vi "Simultaneous Standard.vi"(0 "data server address":string="calcium", 1 "Uncalibrated Index":u32, 2 "Ports":T13) -> ()   [LabVIEW 2012]
uses:
  DAQ configuration/Sensor array.ctl
  DAQ configuration/channel identifier.ctl
  DAC apps/support/method.ctl
  DataServer/command cluster.ctl
  DataServer/command.ctl
  DAC apps/support/Daq state.ctl
  toolbar icons/simultaneous standard cal.ctl
  calib array.ctl
  conversion.ctl
  DAQ configuration/scale type.ctl
  correspondence table.ctl
  pH/pH scale.ctl
  Dissolved Oxygen/DO scale.ctl
  toolbar icons/Save calibration.ctl
  global scale array.vi
panel:
  out "Calibration Graph":cluster{dbl[], dbl[]}[](graph)
  in  "Number of Segments":i32=50
  in  "Save calibration":T1
  out "initial Calibration matrix":T2 {"D.O."."K" format="%.6f"; "D.O."."Temperature" format="%.2f"; "pH scale"."Buffers"."V/T" format="%.5f"; "pH scale"."Buffers"."Buffer" format="%.2f"; "pH scale"."Temperature" format="%.2f"; "offset (physical units)" format="%.5f"; "correspondence table"."volts" format="%.4f"; "correspondence table"."physical units" format="%.4f"; "second channel" min=-1; "offset (volts)" format="%.5f"; "conversion matrix" format="%.4e"}
  in  "Cancel Button":bool
  in  "new daq state":T8
  in  "Acquire Sample":T9
  out "daq state":T8
  in  "Stop acquisition":bool
  in  "Smoothed data frequency":ext=10.0 format="%.4f"
  out "Sampling data frequency":dbl
  in  "method":T10={"sampling interval"=0.1, "samples to average"=1, "data interval"=0.0, "stream data"=FALSE, "file path"=refnum, "command"={"command"=enum."Idle", "start time (ms)"=0, "Channel Indices"=[], "Scans per Sample"=1}} {"command"."Scans per Sample" min=1; "data interval" format="%.2f"; "samples to average" min=1 step=1; "sampling interval" format="%.2f"}
  out "chart":sgl[][](graph)
  out "backlog":u32
  in  "data points to acquire":u32=1000 min=1
  out "error":errorcluster={"status"=FALSE, "code"=56, "source"="TCP Read in \u0000TCP read variable.vi->read Volts data fast.vi->Signal Monitor"}
  in  "OK":bool
  out "units":string
  out "name":string
  in  "Standard\nChannel":i32 min=0 step=1
  # "C"
  # "kPa"
  # "C"
  # "s"
  # "s"
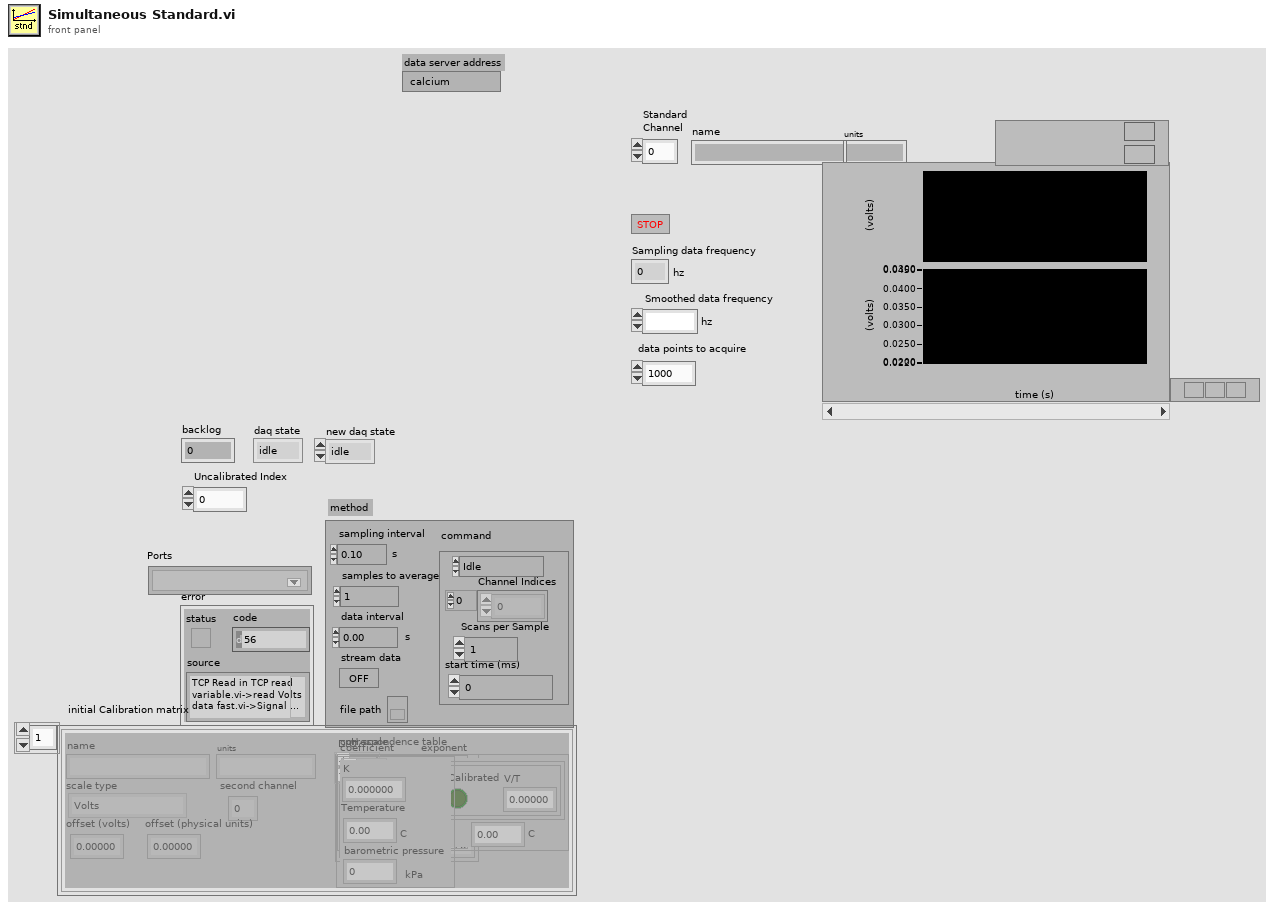
[diagram p1: front panel]
types:
  T1 = typedef "Save calibration.ctl" = bool
  T2 = typedef "calib array.ctl" = T3[]
  T3 = typedef "conversion.ctl" = cluster{"conversion matrix":sgl[][], "units":string, "name":string, "scale type":T4, "offset (volts)":dbl, "second channel":i8, "correspondence table":T5, "offset (physical units)":dbl, "pH scale":T6, "D.O.":T7}
  T4 = typedef "scale type.ctl" = enum16{"Volts", "Polynomial", "Correspondence Table", "pH", "Dissolved Oxygen", "Quadratic"}
  T5 = typedef "correspondence table.ctl" = cluster{"physical units":dbl, "volts":dbl}[]
  T6 = typedef "pH scale.ctl" = cluster{"Buffers":cluster{"Buffer":dbl, "Calibrated":bool, "V/T":dbl}[], "Temperature":dbl}
  T7 = typedef "DO scale.ctl" = cluster{"Temperature":dbl, "K":dbl, "barometric pressure":dbl}
  T8 = typedef "Daq state.ctl" = enum16{"idle", "start", "stream", "clear", "process data", "quit"}
  T9 = typedef "simultaneous standard cal.ctl" = bool
  T10 = typedef "method.ctl" = cluster{"sampling interval":sgl, "samples to average":u32, "data interval":sgl, "stream data":bool, "file path":refnum<file>, "command":T11}
  T11 = typedef "command cluster.ctl" = cluster{"command":T12, "start time (ms)":u32, "Channel Indices":i32[], "Scans per Sample":i32}
  T12 = typedef "command.ctl" = enum16{"Idle", "Send Data", "Send 1 Scan", "Logoff"}
  T13 = typedef "Sensor array.ctl" = T14[]
  T14 = typedef "channel identifier.ctl" = u16
  T15 = enum16{"Idle", "Send Data", "Send 1 Scan", "Logoff"}
  T16 = enum16{"Volts", "Polynomial", "Correspondence Table", "pH", "Dissolved Oxygen"}
  T17 = typedef "Server stats.ctl" = cluster{"scan rate":dbl, "# connections":i32, "channel settings":cluster{"Name":string, "upper input limits":sgl, "lower input limits":sgl, "Location":string}[]}
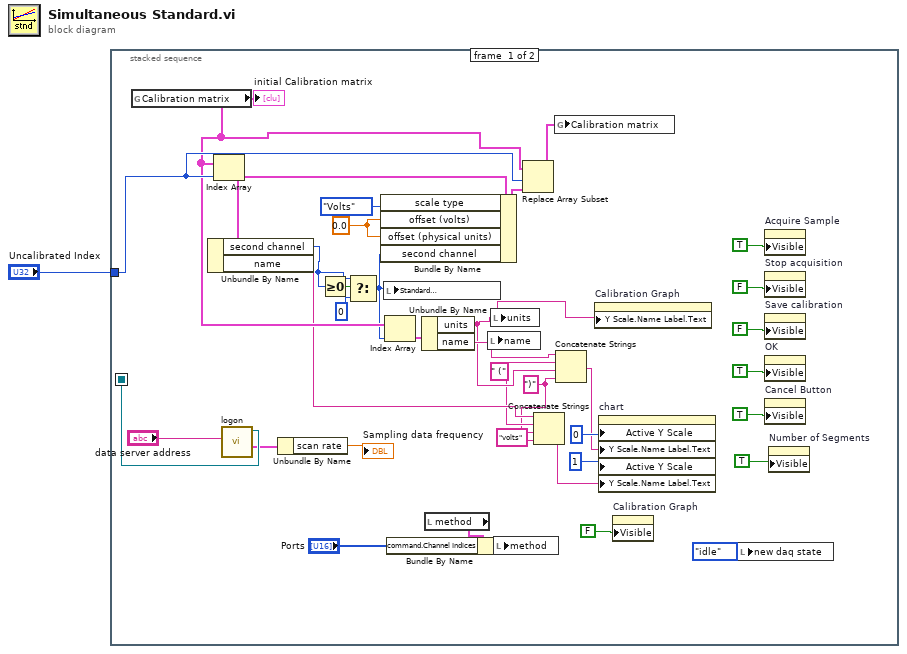
[diagram p0: block diagram]
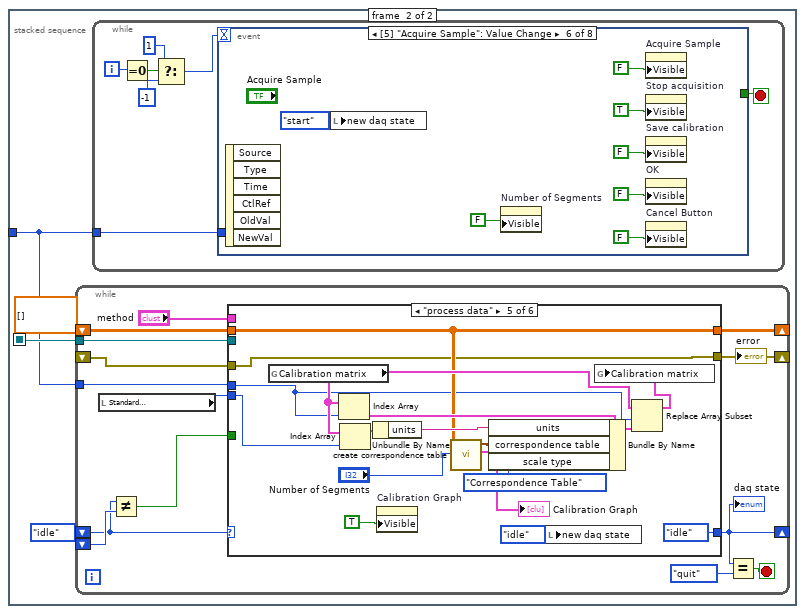
[diagram p2: hidden frame]
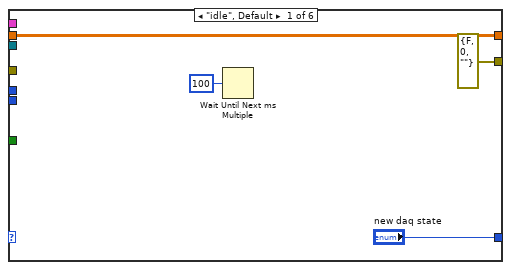
[diagram p3: hidden frame]
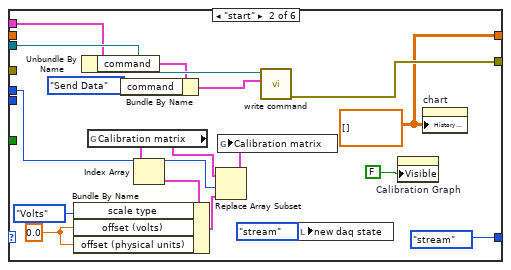
[diagram p4: hidden frame]
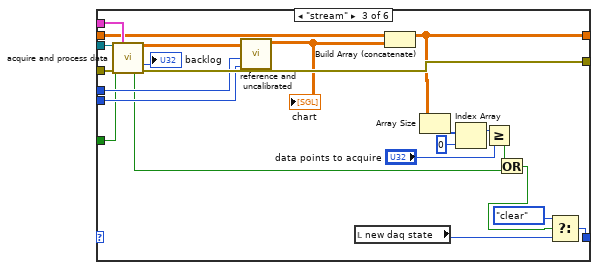
[diagram p5: hidden frame]
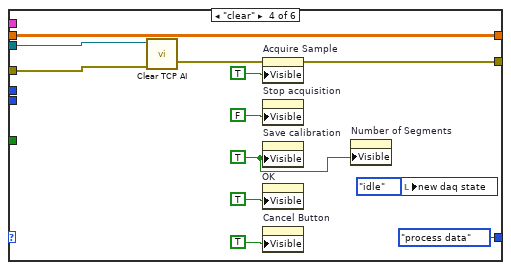
[diagram p6: hidden frame]
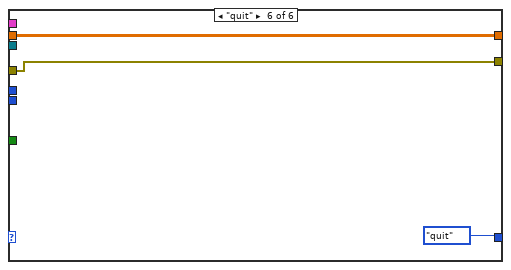
[diagram p7: hidden frame]
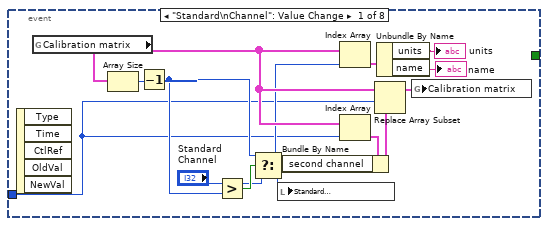
[diagram p8: hidden frame]
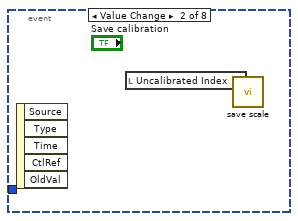
[diagram p9: hidden frame]
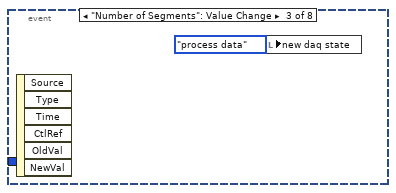
[diagram p10: hidden frame]
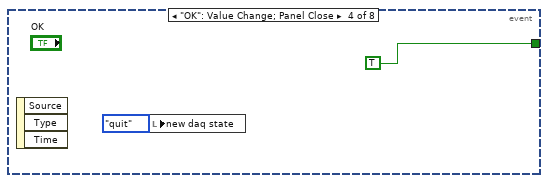
[diagram p11: hidden frame]
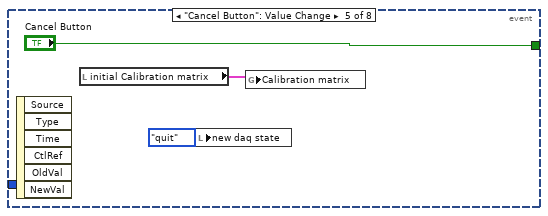
[diagram p12: hidden frame]
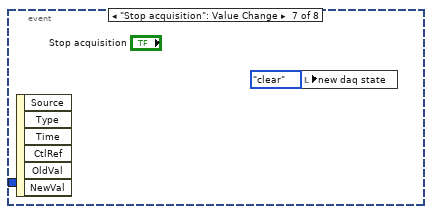
[diagram p13: hidden frame]
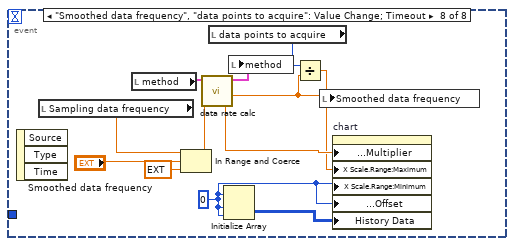
[diagram p14: hidden frame]
diagram:
  n1 = stacked-sequence {
    seq-local: [w5 _] -> [_ w42]
    tunnel: "Uncalibrated Index" -> [w29 w39]
    frame #0 {
      w8 = ")"
      w10 = " ("
      w27 = 0.0 ("offset (volts)")
      n2 = global read "global scale array.vi" "Calibration matrix"() -> (w22:T2)
      "initial Calibration matrix" <- w22
      n3 = Index Array(array=w22, index=w29) -> (element=w21:T3)
      n4 = Unbundle By Name(w21) -> ("second channel"=w20:i8, "name"=w11:string)
      n5 = call "logon.vi"("data server address in"="data server address") -> ("Server stats"=w4:T17, "connection ID"=w5:refnum<k5>)  [unwired: 7 in, 2 out]
      n6 = Unbundle By Name(w4) -> ("scan rate"=→"Sampling data frequency":dbl)
      n7 = Greater Or Equal To 0?(x=w20) -> (x >= 0?=w18:bool)
      n8 = Select(t=w20, s=w18, f=i8 0 ("second channel")) -> (s? t:f=w19:i8)
      n9 = Bundle By Name(cluster=w21, "scale type"=scale_type."Volts", "offset (volts)"=w27, "offset (physical units)"=w27, "second channel"=w19) -> (w30:T3)
      n10 = local write "Standard\nChannel"(w19) -> ()
      n11 = Index Array(array=w22, index=w19) -> (element=w23:T3)
      n12 = Unbundle By Name(w23) -> ("units"=w12:string, "name"=w16:string)
      n13 = local read "method"() -> (w38:T10)
      n14 = Bundle By Name(cluster=w38, "command.Channel Indices"="Ports") -> (w37:T10)
      n15 = local write "name"(w16) -> ()
      n16 = local write "units"(w12) -> ()
      n17 = local write "method"(w37) -> ()
      n18 = Replace Array Subset(array=w22, new element=w30, index=w29) -> (w25:T2)
      n19 = Concatenate Strings(w11, w10, "volts" ("Y Scale.Name Label.Text"), w8) -> (w7:string)
      n20 = global write "global scale array.vi" "Calibration matrix"(w25) -> ()
      n21 = Concatenate Strings(w16, w10, w12, w8) -> (w14:string)
      n22 = property on="Calibration Graph" class="XYGraph (strict)"("Y Scale.Name Label.Text"=w12) -> ()  [unwired: 2 in, 2 out]
      n23 = property on="chart" class="WFChart (strict)"("Active Y Scale"=0, "Y Scale.Name Label.Text"=w14, "Active Y Scale"=1, "Y Scale.Name Label.Text"=w7) -> ()  [unwired: 2 in, 2 out]
      n24 = property on="Calibration Graph" class="XYGraph (strict)"("Visible"=FALSE) -> ()  [unwired: 2 in, 2 out]
      n25 = local write "new daq state"(Daq_state."idle" ("new daq state")) -> ()
      n26 = property on="Acquire Sample" class="Bool"("Visible"=TRUE) -> ()  [unwired: 2 in, 2 out]
      n27 = property on="Stop acquisition" class="Bool"("Visible"=FALSE) -> ()  [unwired: 2 in, 2 out]
      n28 = property on="Save calibration" class="Bool"("Visible"=FALSE) -> ()  [unwired: 2 in, 2 out]
      n29 = property on="OK" class="Bool"("Visible"=TRUE) -> ()  [unwired: 2 in, 2 out]
      n30 = property on="Cancel Button" class="Bool"("Visible"=TRUE) -> ()  [unwired: 2 in, 2 out]
      n31 = property on="Number of Segments" class="DigNum (strict)"("Visible"=TRUE) -> ()  [unwired: 2 in, 2 out]
    }
    frame #1 {
      w40 = Daq_state."idle" ("daq state")
      n32 = while {
        tunnel: w42 -> [w56]
        shift-right: [w54] -> _
        shift-left: sgl[][] [] -> [w53]
        shift-right: [w46] -> _
        shift-left: w40 -> [w48]
        shift-right: [w52] -> _
        shift-left: _ -> [w50]
        tunnel: w39 -> [w51]
        shift-left: w40 -> [w49]
        stop <- w44 stop-if-true
        n33 = local read "Standard\nChannel"() -> (w43:i32)
        n34 = Not Equal?(x=w48, y=w49) -> (x != y?=w47:bool)
        n35 = case shown="\"process data\"" w48 {
          tunnel: [errorcluster {"status"=FALSE, "code"=0, "source"=""} ("error out") w72 w96 w108 w119 w129] -> w52
          tunnel: w50 -> [_ _ w99 w109 w119 w129]
          tunnel: "method" -> [_ w75 w98 _ _ _]
          tunnel: w56 -> [_ w76 w97 w110 _ _]
          tunnel: [w57 w69 w86 w107 w120 w130] -> w54
          tunnel: w53 -> [w57 _ w85 w107 w120 w130]
          tunnel: w51 -> [_ w62 w95 _ w114 _]
          tunnel: w43 -> [_ _ w94 _ w113 _]
          tunnel: w47 -> [_ _ w84 _ _ _]
          tunnel: ["new daq state" Daq_state."stream" ("daq state") w81 Daq_state."process data" ("daq state") Daq_state."idle" ("daq state") Daq_state."quit" ("y")] -> w46
          frame "idle", Default {
            n36 = Wait Until Next ms Multiple(millisecond multiple=u32 100) -> ()  [unwired: 1 out]
          }
          frame "start" {
            w65 = 0.0 ("offset (volts)")
            w69 = sgl[][] []
            n37 = Unbundle By Name(w75) -> ("command"=w74:T11)
            n38 = global read "global scale array.vi" "Calibration matrix"() -> (w67:T2)
            n39 = Bundle By Name(cluster=w74, "command"=T15."Send Data") -> (w77:T11)
            n40 = Index Array(array=w67) -> (element=w63:T3)  [unwired: 1 in]
            n41 = Bundle By Name(cluster=w63, "scale type"=scale_type."Volts", "offset (volts)"=w65, "offset (physical units)"=w65) -> (w68:T3)
            n42 = Replace Array Subset(array=w67, new element=w68, index=w62) -> (w64:T2)
            n43 = global write "global scale array.vi" "Calibration matrix"(w64) -> ()
            n44 = call "write command.vi"("command interface"=w77, "refnum in"=w76) -> ("error out"=w72:errorcluster)  [unwired: 8 in, 1 out]
            n45 = local write "new daq state"(Daq_state."stream" ("new daq state")) -> ()
            n46 = property on="Calibration Graph" class="XYGraph (strict)"("Visible"=FALSE) -> ()  [unwired: 2 in, 2 out]
            n47 = property on="chart" class="WFChart (strict)"("History Data"=w69) -> ()  [unwired: 2 in, 2 out]
          }
          frame "stream" {
            n48 = call "acquire and process data.vi"("connection ID"=w97, "Reset"=w84, "error in"=w99, "method"=w98) -> ("data out"=w87:sgl[][], "backlog"=→"backlog":u32, "Status"=w79:bool, "error out"=w96:errorcluster)  [unwired: 4 in, 4 out]
            n49 = call "reference and uncalibrated.vi"("Reference Index"=w94, "uncalibrated index"=w95, "scaled data"=w87) -> ("reference and volts"=w78:sgl[][])  [unwired: 4 in]
            "chart" <- w78
            n50 = local read "new daq state"() -> (w80:T8)
            n51 = Build Array (concatenate)(w85, w78) -> (w86:sgl[][])
            n52 = Array Size(array=w86) -> (size(s)=w92:i32[])
            n53 = Index Array(array=w92, index=0 ("Index")) -> (element=w90:i32)
            n54 = Greater Or Equal?(x=w90, y="data points to acquire") -> (x >= y?=w88:bool)
            n55 = Or(x=w88, y=w79) -> (x .or. y?=w82:bool)
            n56 = Select(t=Daq_state."clear" ("daq state"), s=w82, f=w80) -> (s? t:f=w81:T8)
          }
          frame "clear" {
            w100 = TRUE ("Visible")
            n57 = call "Clear TCP AI.vi"("error in (no error)"=w109, "Connection ID in"=w110) -> ("error out"=w108:errorcluster)  [unwired: 8 in, 1 out]
            n58 = property on="Acquire Sample" class="Bool"("Visible"=TRUE) -> ()  [unwired: 2 in, 2 out]
            n59 = property on="Stop acquisition" class="Bool"("Visible"=FALSE) -> ()  [unwired: 2 in, 2 out]
            n60 = property on="Save calibration" class="Bool"("Visible"=w100) -> ()  [unwired: 2 in, 2 out]
            n61 = property on="OK" class="Bool"("Visible"=TRUE) -> ()  [unwired: 2 in, 2 out]
            n62 = property on="Cancel Button" class="Bool"("Visible"=TRUE) -> ()  [unwired: 2 in, 2 out]
            n63 = property on="Number of Segments" class="DigNum (strict)"("Visible"=w100) -> ()  [unwired: 2 in, 2 out]
            n64 = local write "new daq state"(Daq_state."idle" ("new daq state")) -> ()
          }
          frame "process data" {
            n65 = global read "global scale array.vi" "Calibration matrix"() -> (w123:T2)
            n66 = Index Array(array=w123, index=w114) -> (element=w124:T3)
            n67 = Index Array(array=w123, index=w113) -> (element=w122:T3)
            n68 = Unbundle By Name(w122) -> ("units"=w121:string)
            n69 = property on="Calibration Graph" class="XYGraph (strict)"("Visible"=TRUE) -> ()  [unwired: 2 in, 2 out]
            n70 = call "create correspondence table.vi"("pieces"="Number of Segments", "data array"=w120) -> ("calibration graph"=→"Calibration Graph":cluster{dbl[], dbl[]}[], "correspondence table"=w115:T5)  [unwired: 8 in]
            n71 = Bundle By Name(cluster=w124, "units"=w121, "correspondence table"=w115, "scale type"=T16."Correspondence Table" ("Bundle Element")) -> (w126:T3)
            n72 = local write "new daq state"(Daq_state."idle" ("new daq state")) -> ()
            n73 = Replace Array Subset(array=w123, new element=w126, index=w114) -> (w127:T2)
            n74 = global write "global scale array.vi" "Calibration matrix"(w127) -> ()
          }
          frame "quit" {
          }
        }
        "error" <- w52
        "daq state" <- w46
        n75 = Equal?(x=w46, y=Daq_state."quit") -> (x = y?=w44:bool)
      }
      n76 = while {
        tunnel: w39 -> [w137]
        i -> [w135]
        stop <- w136 stop-if-true
        n77 = Equal To 0?(x=w135) -> (x = 0?=w134:bool)
        n78 = Select(t=1, s=w134, f=-1) -> (s? t:f=w131:i32)
        n79 = event shown="[5] \"Acquire Sample\": Value Change" {
          selector: _ -> [_ _ _ _ _ _ _ _]
          dyn-events: _ -> [_ _ _ _ _ _ _ _]
          timeout: w131 -> [_ _ _ _ _ _ _ _]
          tunnel: w137 -> [w138 _ _ _ _ _ _ _]
          tunnel: [_ _ _ TRUE ("OK") "Cancel Button" _ _ _] -> w136
          event "Standard\nChannel": Value Change {
            n80 = event-data() -> ()  [unwired: 1 in, 5 out]
            n81 = global read "global scale array.vi" "Calibration matrix"() -> (w142:T2)
            n82 = Array Size(array=w142) -> (size(s)=w145:i32)
            n83 = Decrement(x=w145) -> (x-1=w143:i32)
            n84 = Greater?(x="Standard\nChannel", y=w143) -> (0:w144:bool)
            n85 = Select(t=w143, s=w144, f="Standard\nChannel") -> (s? t:f=w140:i32)
            n86 = local write "Standard\nChannel"(w140) -> ()
            n87 = Index Array(array=w142, index=w140) -> (element=w150:T3)
            n88 = Index Array(array=w142, index=w138) -> (element=w149:T3)
            n89 = Bundle By Name(cluster=w149, "second channel"=w140) -> (w148:T3)
            n90 = Replace Array Subset(array=w142, new element=w148, index=w138) -> (w139:T2)
            n91 = Unbundle By Name(w150) -> ("units"=→"units":string, "name"=→"name":string)
            n92 = global write "global scale array.vi" "Calibration matrix"(w139) -> ()
          }
          event Value Change {
            n93 = event-data() -> ()  [unwired: 1 in, 5 out]
            n94 = local read "Uncalibrated Index"() -> (w151:u32)
            n95 = call "save scale.vi"("Index"=w151) -> ()  [unwired: 6 in, 1 out]
          }
          event "Number of Segments": Value Change {
            n96 = event-data() -> ()  [unwired: 1 in, 6 out]
            n97 = local write "new daq state"(Daq_state."process data" ("new daq state")) -> ()
          }
          event "OK": Value Change; Panel Close {
            n98 = event-data() -> ()  [unwired: 1 in, 3 out]
            n99 = local write "new daq state"(Daq_state."quit" ("new daq state")) -> ()
          }
          event "Cancel Button": Value Change {
            n100 = event-data() -> ()  [unwired: 1 in, 6 out]
            n101 = local read "initial Calibration matrix"() -> (w157:T2)
            n102 = local write "new daq state"(Daq_state."quit" ("new daq state")) -> ()
            n103 = global write "global scale array.vi" "Calibration matrix"(w157) -> ()
          }
          event Value Change {
            n104 = event-data() -> ()  [unwired: 1 in, 6 out]
            n105 = local write "new daq state"(Daq_state."start" ("new daq state")) -> ()
            n106 = property on="Number of Segments" class="DigNum (strict)"("Visible"=FALSE) -> ()  [unwired: 2 in, 2 out]
            n107 = property on="Acquire Sample" class="Bool"("Visible"=FALSE) -> ()  [unwired: 2 in, 2 out]
            n108 = property on="Stop acquisition" class="Bool"("Visible"=TRUE) -> ()  [unwired: 2 in, 2 out]
            n109 = property on="Save calibration" class="Bool"("Visible"=FALSE) -> ()  [unwired: 2 in, 2 out]
            n110 = property on="OK" class="Bool"("Visible"=FALSE) -> ()  [unwired: 2 in, 2 out]
            n111 = property on="Cancel Button" class="Bool"("Visible"=FALSE) -> ()  [unwired: 2 in, 2 out]
          }
          event "Stop acquisition": Value Change {
            n112 = event-data() -> ()  [unwired: 1 in, 6 out]
            n113 = local write "new daq state"(Daq_state."clear" ("new daq state")) -> ()
          }
          event "Smoothed data frequency", "data points to acquire": Value Change; Timeout {
            w166 = 0
            n114 = event-data() -> ()  [unwired: 1 in, 3 out]
            n115 = local read "Sampling data frequency"() -> (w176:dbl)
            n116 = local read "method"() -> (w172:T10)
            n117 = In Range and Coerce(upper limit=w176, x="Smoothed data frequency", lower limit=ext 0.01) -> (coerced(x)=w173:ext)  [unwired: 1 out]
            n118 = call "data rate calc.vi"("Data frequency"=w173, "method in"=w172) -> ("new data interval"=w171:sgl, "new data frequency"=w168:ext, "method out"=w177:T10)  [unwired: 2 in, 1 out]
            n119 = local read "data points to acquire"() -> (w169:u32)
            n120 = Initialize Array(w166, w166, w166) -> (w170:i32[][])
            n121 = local write "method"(w177) -> ()
            n122 = Divide(x=w169, y=w168) -> (x/y=w167:ext)
            n123 = local write "Smoothed data frequency"(w168) -> ()
            n124 = property on="chart" class="WFChart (strict)"("X Scale.Offset and Multiplier:Multiplier"=w171, "X Scale.Range:Maximum"=w167, "X Scale.Range:Minimum"=w166, "X Scale.Offset and Multiplier:Offset"=w166, "History Data"=w170) -> ()  [unwired: 2 in, 2 out]
          }
        }
      }
    }
  }
